vi "DAC Run.vi"(8 "error in":errorcluster, 11 "DAC Inclino in":refnum<class "DAC Inclinometer.lvclass">) -> (0 "error out":errorcluster, 3 "DAC Inclino out":refnum<class "DAC Inclinometer.lvclass">)   [LabVIEW 2019, in "DAC.lvlib" / "DAC Inclinometer.lvclass"]
uses:
  DAC Inclinometer.lvclass
  C:/Users/wg/Documents/LV_Projects/test-stand/App/DAC/DAC.lvclass
  DAC.lvclass/DAC.ctl
  Results/Results Method.ctl
  Results/Water Tunnel Results/Water Tunnel Results.lvclass
  DAC Inclinometer.lvclass/DAC Inclinometer.ctl
  Results/Water Tunnel Results/Water Tunnel Results.lvclass/Water Tunnel Results.ctl
  <vilib>/DAQmx/read.llb/DAQmx Read (Analog DBL 1Chan 1Samp).vi
  <vilib>/DAQmx/miscellaneous.llb/DAQmx Fill In Error Info.vi
  DAC.lvclass
  Results/Results.lvlib
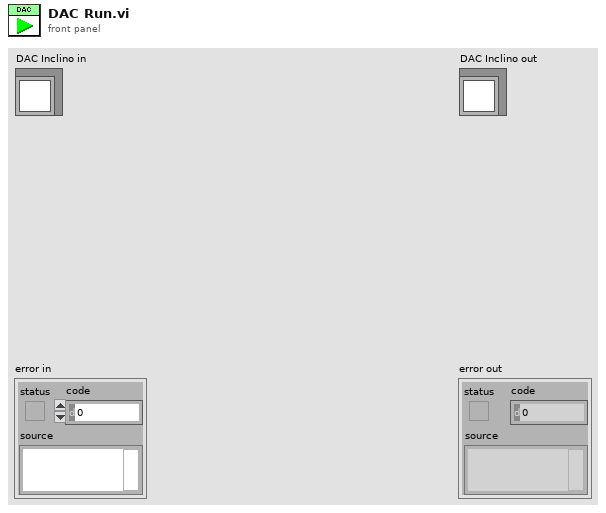
[diagram p1: front panel]
types:
  T1 = typedef "Results.lvlib/Results Method.ctl" = enum16{"Get", "Set"}
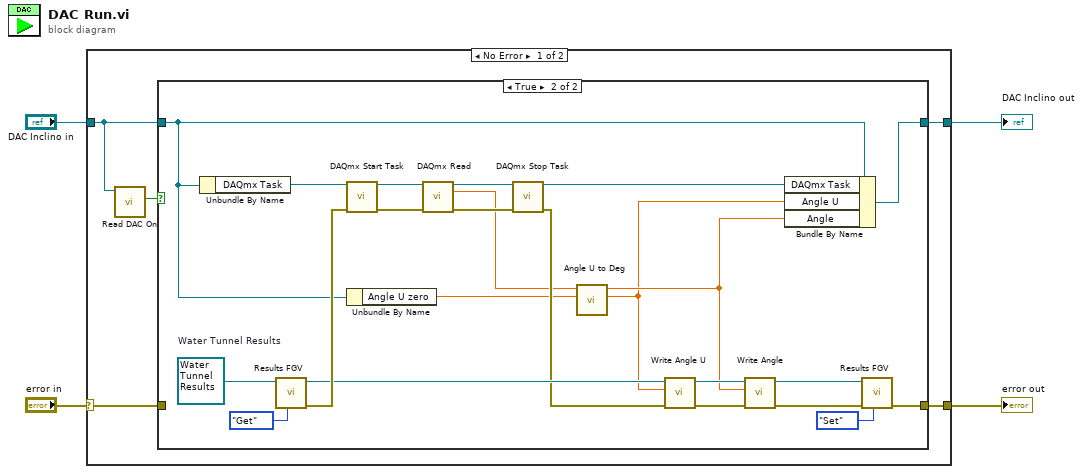
[diagram p0: block diagram]
diagram:
  n1 = case shown="No Error" "error in" {
    selector: "error in" -> [w7 w36]
    tunnel: [w6 w36] -> w2
    tunnel: [w8 w35] -> w1
    tunnel: "DAC Inclino in" -> [w5 w35]
    frame No Error {
      n2 = call "Read DAC On.vi"("DAC in"=w5) -> ("DAC On"=w9:bool)  [unwired: 8 in, 2 out]
      n3 = case shown="True" w9 {
        tunnel: w5 -> [w11 w22]
        tunnel: [w11 w25] -> w8
        tunnel: w7 -> [w10 _]
        tunnel: [w10 w24] -> w6
        frame False {
        }
        frame True {
          w23 = refnum<class "Water Tunnel Results.lvclass"> refnum  # Water Tunnel Results
          n4 = Unbundle By Name(w22) -> ("DAQmx Task"=w34:refnum<k21>)
          n5 = call-dynamic "Results FGV.vi"("Method"=Results_Method."Get", "Water Tunnel Results in"=w23) -> ("error out"=w28:errorcluster, "Water Tunnel  Results out"=w20:refnum<class "Water Tunnel Results.lvclass">)  [unwired: 8 in]
          n6 = call <vilib>:"DAQmx Start Task.vi"("task/channels in"=w34, "error in"=w28) -> ("task out"=w33:refnum<k21>, "error out"=w32:errorcluster)  [unwired: 12 in]
          n7 = Unbundle By Name(w22) -> ("Angle U zero"=w15:dbl)
          n8 = call-poly <vilib>:"DAQmx Read.vi"("task/channels in"=w33, "error in"=w32) -> ("task out"=w26:refnum<k21>, "data"=w14:dbl, "error out"=w31:errorcluster)  [unwired: 11 in]
          n9 = call <vilib>:"DAQmx Stop Task.vi"("task/channels in"=w26, "error in"=w31) -> ("task out"=w27:refnum<k21>, "error out"=w18:errorcluster)  [unwired: 12 in]
          n10 = call "Angle U to Deg.vi"("Angle U zero"=w15, "Angle U"=w14) -> ("Angle U"=w12:dbl, "Angle"=w13:dbl)  [unwired: 8 in]
          n11 = call "Write Angle U.vi"("error in (no error)"=w18, "Angle U"=w12, "Water Tunnel Results in"=w20) -> ("error out"=w17:errorcluster, "Water Tunnel Results out"=w19:refnum<class "Water Tunnel Results.lvclass">)  [unwired: 7 in]
          n12 = call "Write Angle.vi"("error in (no error)"=w17, "Angle"=w13, "Water Tunnel Results in"=w19) -> ("error out"=w16:errorcluster, "Water Tunnel Results out"=w21:refnum<class "Water Tunnel Results.lvclass">)  [unwired: 7 in]
          n13 = Bundle By Name(cluster=w22, "DAQmx Task"=w27, "Angle U"=w12, "Angle"=w13) -> (w25:refnum<class "DAC Inclinometer.lvclass">)
          n14 = call-dynamic "Results FGV.vi"("Method"=Results_Method."Set", "error in"=w16, "Water Tunnel Results in"=w21) -> ("error out"=w24:errorcluster)  [unwired: 7 in, 1 out]
        }
      }
    }
    frame Error {
    }
  }
  "error out" <- w2
  "DAC Inclino out" <- w1
